vi "Refresh Remote Systems Layout.vi"(8 "error in (no error)":errorcluster, 10 "Draw Area Size":T1, 11 "Editor Handler in":refnum<class "Image Editor Handler.lvclass">) -> (0 "error out":errorcluster)   [LabVIEW 2016]
uses:
  <vilib>/Utility/miscctls.llb/LVBoundsTypeDef.ctl
  <vilib>/LIEF/Image Editor Handler/Image Editor Handler.lvclass
  <vilib>/LIEF/Forms/Grid/Grid.lvclass
  <vilib>/LIEF/Forms/Shape/Shape.lvclass
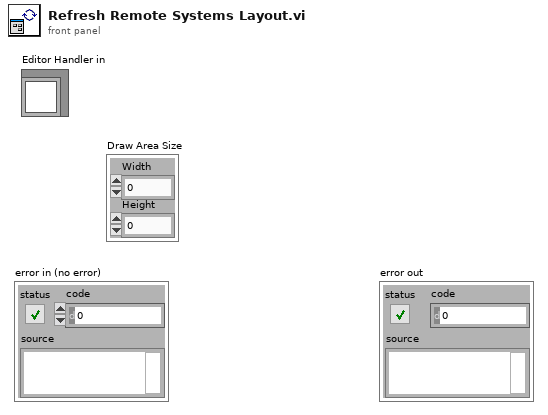
[diagram p1: front panel]
types:
  T1 = typedef "LVBoundsTypeDef.ctl" = cluster{"Width":u32, "Height":u32}
  T2 = enum16{"Left", "Top", "Right", "Bottom", "Centered"}
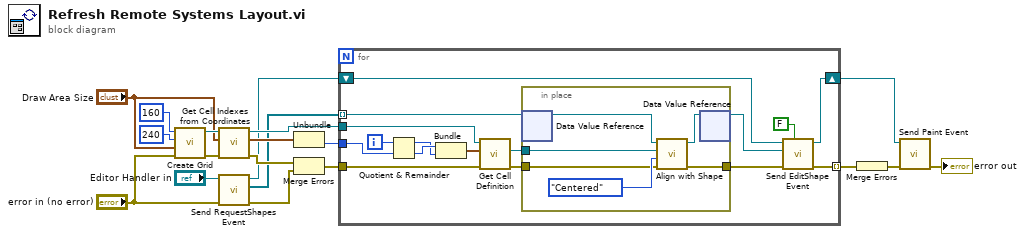
[diagram p0: block diagram]
diagram:
  n1 = call <vilib>:"Create Grid.vi"("error in (no error)"="error in (no error)", "Draw Area"="Draw Area Size", "Horizontal Step"=240, "Vertical Step"=160) -> ("error out"=w10:errorcluster, "Grid Reference"=w12:refnum<data-value>)  [unwired: 6 in]
  n2 = call <vilib>:"Get Cell Indexes from Coordinates.vi"("error in (no error)"=w10, "Coordinates"="Draw Area Size", "Shape Reference"=w12) -> ("error out"=w15:errorcluster, "Indexes"=w18:cluster{"Row":u32, "Column":u32}, "Shape Reference 2"=w16:refnum<data-value>)  [unwired: 6 in]
  n3 = call <vilib>:"Send RequestShapes Event.vi"("error in (no error)"="error in (no error)", "Editor Handler in"="Editor Handler in") -> ("error out"=w3:errorcluster, "Shapes"=w7:refnum<data-value>[], "Editor Handler out"=w6:refnum<class "Image Editor Handler.lvclass">)  [unwired: 7 in]
  n4 = Unbundle(w18) -> ("Column"=w17:u32)  [unwired: 1 out]
  n5 = Merge Errors(w15, w3) -> (w4:errorcluster)
  n6 = for {
    tunnel: [w21] -> w19 mode=indexing
    tunnel: w17 -> [w34]
    tunnel: w16 -> [w31]
    tunnel: w4 -> [w28]
    tunnel: w7 -> [w27] mode=indexing
    shift-right: [w25] -> w9
    shift-left: w6 -> [w24]
    i -> [w35]
    n7 = Quotient & Remainder(x=w35, y=w34) -> (x-y*floor(x/y)=w32:u32, floor(x/y)=w33:u32)
    n8 = Bundle(w33, w32) -> (w30:cluster{u32, u32})  [unwired: 1 in]
    n9 = call <vilib>:"Get Cell Definition.vi"("error in (no error)"=w28, "Indexes"=w30, "Shape Reference"=w31) -> ("error out"=w20:errorcluster, "Cell"=w29:refnum<class "Shape.lvclass">)  [unwired: 6 in, 1 out]
    n10 = in-place {
      in-place-border: w29 -> [w40]
      in-place-border: [w39] -> w22
      in-place-border: w20 -> [w36]
      n11 = in-place-dvr #1(w27) -> (w38:refnum<class "Shape.lvclass">)  [unwired: 1 out]
      n12 = call <vilib>:"Align with Shape.vi"("error in (no error)"=w36, "Alignment"=T2."Centered", "Reference Shape"=w40, "Shape in"=w38) -> ("error out"=w39:errorcluster, "Shape out"=w37:refnum<class "Shape.lvclass">)  [unwired: 6 in]
      n13 = in-place-dvr #1(w37) -> (w23:refnum<data-value>)  [unwired: 1 out]
    }
    n14 = call <vilib>:"Send EditShape Event.vi"("Auto-Refresh (T)"=FALSE, "error in (no error)"=w22, "Shape"=w23, "Editor Handler in"=w24) -> ("error out"=w21:errorcluster, "Editor Handler out"=w25:refnum<class "Image Editor Handler.lvclass">)  [unwired: 6 in]
  }
  n15 = Merge Errors(w19) -> (w2:errorcluster)
  n16 = call <vilib>:"Send Paint Event.vi"("error in (no error)"=w2, "Editor Handler in"=w9) -> ("error out"=→"error out":errorcluster)  [unwired: 8 in, 1 out]
